vi "PingTestBoard(LC).vi"(0 "COMPORT":refnum<visa-resource-name>, 2 "GuiDir":path, 3 "GlobPaths(t)":bool=TRUE, 5 "error in (no error)":errorcluster, 7 "Mode Select":i32(ring) items=["CW", "DYNAMIC"], 9 "Close Serial(T)":bool, 11 "ExeCommands(T)":bool, 13 "RevC(t)":bool) -> (8 "standard error":string, 10 "standard output":string="Server Status Ok. Received 2048 samples\r\n", 12 "OK?(t)":bool=TRUE, 14 "Run_DMI(t)":bool, 15 "Run_AMInit(t)":bool, 17 "Run -dyn(t)":bool, 19 "error out":errorcluster)   [LabVIEW 2018]
uses:
  Initialize References/Sequence Globals.vi
panel:
  out "ping":string
  out "py_com_port":string
  out "Numeric":i32
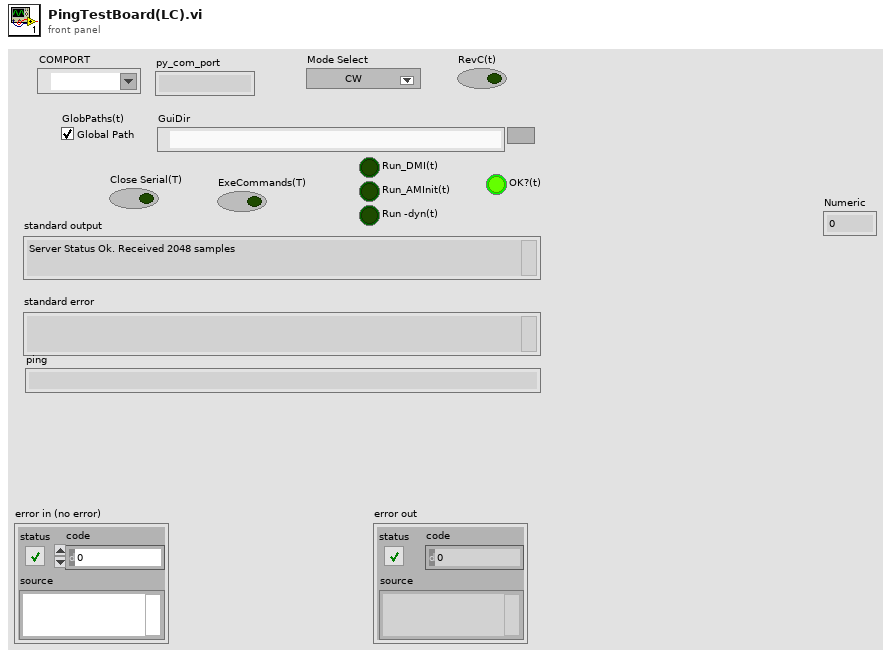
[diagram p1: front panel]
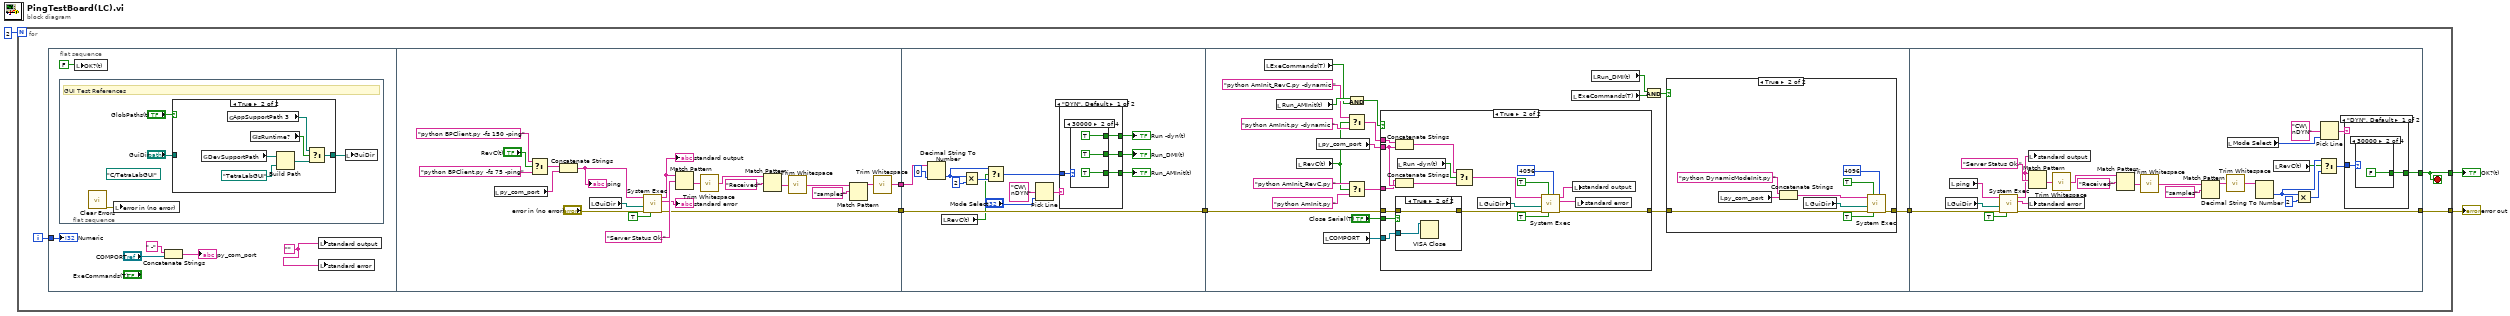
[diagram p0: block diagram]
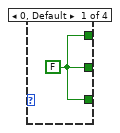
[diagram p3: hidden frame]
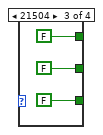
[diagram p4: hidden frame]
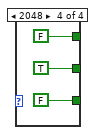
[diagram p5: hidden frame]
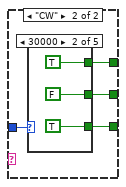
[diagram p6: hidden frame]
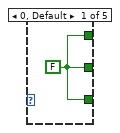
[diagram p7: hidden frame]
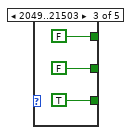
[diagram p8: hidden frame]
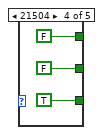
[diagram p9: hidden frame]
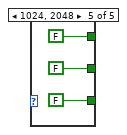
[diagram p10: hidden frame]
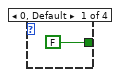
[diagram p14: hidden frame]
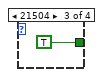
[diagram p15: hidden frame]
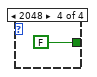
[diagram p16: hidden frame]
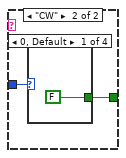
[diagram p17: hidden frame]
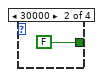
[diagram p18: hidden frame]
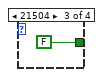
[diagram p19: hidden frame]
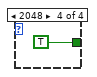
[diagram p20: hidden frame]
diagram:
  n1 = for {
    N: 2 -> [_]
    tunnel: [w6] -> w3
    tunnel: [w5] -> w2
    i -> [w4]
    stop <- w5 stop-if-true
    n2 = flat-sequence {
      tunnel: w4 -> [w12]
      tunnel: [w39] -> w10
      tunnel: [w38] -> w9
      tunnel: w10 -> [w55]
      tunnel: [w58] -> w8
      tunnel: w9 -> [w58]
      tunnel: w8 -> [w112]
      tunnel: [w110] -> w7
      tunnel: [w156] -> w6
      tunnel: w7 -> [w157]
      tunnel: [w153] -> w5
      frame #0 {
        w11 = ""
        n3 = flat-sequence {
          frame #0 {
            (unwired) path "C:/TetraLabGUI" ("PyScript(path)")
            # "GUI Test References"
            n4 = call <vilib>:"Clear Errors.vi"() -> ("error out"=w19:errorcluster)  [unwired: 6 in, 1 out]
            n5 = local write "error in (no error)"(w19) -> ()
            n6 = case shown="True" "GlobPaths(t)" {
              tunnel: [w21 w25] -> w20
              tunnel: "GuiDir" -> [w21 _]
              frame False {
              }
              frame True {
                n7 = global read "Sequence Globals.vi" "DevSupportPath"() -> (w24:path)
                n8 = global read "Sequence Globals.vi" "AppSupportPath 3"() -> (w26:path)
                n9 = global read "Sequence Globals.vi" "IsRuntime?"() -> (w27:bool)
                n10 = Build Path(base path=w24, name or relative path=path "TetraLabGUI" ("PyScript(path)")) -> (appended path=w22:path)
                n11 = Select(t=w26, s=w27, f=w22) -> (s? t:f=w25:path)
              }
            }
            n12 = local write "GuiDir"(w20) -> ()
          }
        }
        n13 = local write "OK?(t)"(FALSE ("OK?(t)")) -> ()
        n14 = Concatenate Strings(" -" ("string"), "COMPORT") -> (→"py_com_port":string)
        n15 = local write "standard output"(w11) -> ()
        n16 = local write "standard error"(w11) -> ()
        "Numeric" <- w12
      }
      frame #1 {
        n17 = local read "py_com_port"() -> (w32:string)
        n18 = Select(t="python BPClient.py -fs 150 -ping" ("command line"), s="RevC(t)", f="python BPClient.py -fs 75 -ping" ("command line")) -> (s? t:f=w31:string)
        n19 = Concatenate Strings(w31, w32) -> (w33:string)
        "ping" <- w33
        n20 = local read "GuiDir"() -> (w34:path)
        n21 = call <vilib>:"System Exec.vi"("run minimized? (F)"=TRUE, "error in (no error)"="error in (no error)", "working directory"=w34, "command line"=w33) -> ("error out"=w38:errorcluster, "standard error"=→"standard error":string, "standard output"=w48:string)  [unwired: 4 in, 1 out]
        "standard output" <- w48
        n22 = Match Pattern(string=w48, regular expression="Server Status Ok.") -> (after substring=w43:string)  [unwired: 1 in, 3 out]
        n23 = call <vilib>:"Trim Whitespace.vi"("string"=w43) -> ("trimmed string"=w44:string)  [unwired: 1 in]
        n24 = Match Pattern(string=w44, regular expression="Received") -> (after substring=w45:string)  [unwired: 1 in, 3 out]
        n25 = call <vilib>:"Trim Whitespace.vi"("string"=w45) -> ("trimmed string"=w47:string)  [unwired: 1 in]
        n26 = Match Pattern(string=w47, regular expression="samples") -> (before substring=w46:string)  [unwired: 1 in, 3 out]
        n27 = call <vilib>:"Trim Whitespace.vi"("string"=w46) -> ("trimmed string"=w39:string)  [unwired: 1 in]
      }
      frame #2 {
        n28 = Decimal String To Number(string=w55, default (0L)=i16 0 ("default (0 I32)")) -> (number=w52:i16)  [unwired: 1 in, 1 out]
        n29 = local read "RevC(t)"() -> (w49:bool)
        n30 = Multiply(x=w52, y=i16 2) -> (x*y=w53:i16)
        n31 = Select(t=w52, s=w49, f=w53) -> (s? t:f=w50:i16)
        n32 = Pick Line(multi-line string="CW\nDYN", line index="Mode Select") -> (output string=w61:string)  [unwired: 1 in]
        n33 = case shown="\"DYN\", Default" w61 {
          tunnel: w50 -> [w66 w80]
          tunnel: [w65 w79] -> w56
          tunnel: [w64 w78] -> w59
          tunnel: [w63 w77] -> w57
          frame "DYN", Default {
            n34 = case shown="30000" w66 {
              tunnel: [w67 TRUE FALSE TRUE] -> w65
              tunnel: [w67 TRUE FALSE FALSE] -> w64
              tunnel: [w67 TRUE FALSE FALSE] -> w63
              frame 0, Default {
                w67 = FALSE
              }
              frame 30000 {
              }
              frame 21504 {
              }
              frame 2048 {
              }
            }
          }
          frame "CW" {
            n35 = case shown="30000" w80 {
              tunnel: [w81 FALSE FALSE FALSE FALSE] -> w79
              tunnel: [w81 TRUE TRUE TRUE FALSE] -> w78
              tunnel: [w81 TRUE FALSE FALSE FALSE] -> w77
              frame 0, Default {
                w81 = FALSE
              }
              frame 30000 {
              }
              frame 2049..21503 {
              }
              frame 21504 {
              }
              frame 1024, 2048 {
              }
            }
          }
        }
        "Run_DMI(t)" <- w56
        "Run_AMInit(t)" <- w59
        "Run -dyn(t)" <- w57
      }
      frame #3 {
        n36 = local read "ExeCommands(T)"() -> (w104:bool)
        n37 = local read "Run_AMInit(t)"() -> (w105:bool)
        n38 = local read "RevC(t)"() -> (w94:bool)
        n39 = local read "py_com_port"() -> (w101:string)
        n40 = local read "COMPORT"() -> (w102:refnum<visa-resource-name>)
        n41 = And(x=w105, y=w104) -> (x .and. y?=w109:bool)
        n42 = Select(t="python AmInit_RevC.py -dynamic " ("command line"), s=w94, f="python AmInit.py -dynamic " ("command line")) -> (s? t:f=w98:string)
        n43 = Select(t="python AmInit_RevC.py " ("command line"), s=w94, f="python AmInit.py " ("command line")) -> (s? t:f=w95:string)
        n44 = case shown="True" w109 {
          tunnel: w112 -> [w123 w136]
          tunnel: [w123 w138] -> w111
          tunnel: w102 -> [_ w134]
          tunnel: "Close Serial(T)" -> [_ w133]
          tunnel: w101 -> [_ w129]
          tunnel: w98 -> [_ w128]
          tunnel: w95 -> [_ w127]
          frame False {
          }
          frame True {
            n45 = Concatenate Strings(w128, w129) -> (w131:string)
            n46 = Concatenate Strings(w127, w129) -> (w130:string)
            n47 = case shown="True" w133 {
              tunnel: w136 -> [w142 w143]
              tunnel: [w142 w143] -> w135
              tunnel: w134 -> [_ w144]
              frame False {
              }
              frame True {
                n48 = VISA Close(VISA resource name=w144) -> ()  [unwired: 1 in, 1 out]
              }
            }
            n49 = local read "Run -dyn(t)"() -> (w137:bool)
            n50 = Select(t=w131, s=w137, f=w130) -> (s? t:f=w126:string)
            n51 = local read "GuiDir"() -> (w132:path)
            n52 = call <vilib>:"System Exec.vi"("expected output size  (4096)"=u32 4096, "run minimized? (F)"=TRUE, "wait until completion? (T)"=TRUE, "error in (no error)"=w135, "working directory"=w132, "command line"=w126) -> ("error out"=w138:errorcluster, "standard error"=w125:string, "standard output"=w124:string)  [unwired: 2 in, 1 out]
            n53 = local write "standard output"(w124) -> ()
            n54 = local write "standard error"(w125) -> ()
          }
        }
        n55 = local read "ExeCommands(T)"() -> (w106:bool)
        n56 = local read "Run_DMI(t)"() -> (w107:bool)
        n57 = And(x=w107, y=w106) -> (x .and. y?=w108:bool)
        n58 = case shown="True" w108 {
          tunnel: [w113 w121] -> w110
          tunnel: w111 -> [w113 w118]
          frame False {
          }
          frame True {
            n59 = local read "py_com_port"() -> (w114:string)
            n60 = Concatenate Strings("python DynamicModeInit.py " ("command line"), w114) -> (w115:string)
            n61 = local read "GuiDir"() -> (w116:path)
            n62 = call <vilib>:"System Exec.vi"("expected output size  (4096)"=u32 4096, "run minimized? (F)"=TRUE, "wait until completion? (T)"=TRUE, "error in (no error)"=w118, "working directory"=w116, "command line"=w115) -> ("error out"=w121:errorcluster)  [unwired: 2 in, 3 out]
          }
        }
      }
      frame #4 {
        n63 = local read "GuiDir"() -> (w152:path)
        n64 = local read "ping"() -> (w145:string)
        n65 = call <vilib>:"System Exec.vi"("run minimized? (F)"=TRUE, "error in (no error)"=w157, "working directory"=w152, "command line"=w145) -> ("error out"=w156:errorcluster, "standard error"=w154:string, "standard output"=w155:string)  [unwired: 4 in, 1 out]
        n66 = local write "standard output"(w155) -> ()
        n67 = Match Pattern(string=w155, regular expression="Server Status Ok.") -> (after substring=w164:string)  [unwired: 1 in, 3 out]
        n68 = local write "standard error"(w154) -> ()
        n69 = call <vilib>:"Trim Whitespace.vi"("string"=w164) -> ("trimmed string"=w165:string)  [unwired: 1 in]
        n70 = Match Pattern(string=w165, regular expression="Received") -> (after substring=w166:string)  [unwired: 1 in, 3 out]
        n71 = call <vilib>:"Trim Whitespace.vi"("string"=w166) -> ("trimmed string"=w168:string)  [unwired: 1 in]
        n72 = Match Pattern(string=w168, regular expression="samples") -> (before substring=w167:string)  [unwired: 1 in, 3 out]
        n73 = call <vilib>:"Trim Whitespace.vi"("string"=w167) -> ("trimmed string"=w151:string)  [unwired: 1 in]
        n74 = local read "Mode Select"() -> (w169:i32)
        n75 = Decimal String To Number(string=w151) -> (number=w148:i32)  [unwired: 2 in, 1 out]
        n76 = local read "RevC(t)"() -> (w146:bool)
        n77 = Multiply(x=w148, y=2) -> (x*y=w149:i32)
        n78 = Select(t=w148, s=w146, f=w149) -> (s? t:f=w150:i32)
        n79 = Pick Line(multi-line string="CW\nDYN", line index=w169) -> (output string=w163:string)  [unwired: 1 in]
        n80 = case shown="\"DYN\", Default" w163 {
          tunnel: w150 -> [w171 w177]
          tunnel: [w170 w176] -> w153
          frame "DYN", Default {
            n81 = case shown="30000" w171 {
              tunnel: [FALSE FALSE TRUE FALSE] -> w170
              frame 0, Default {
              }
              frame 30000 {
              }
              frame 21504 {
              }
              frame 2048 {
              }
            }
          }
          frame "CW" {
            n82 = case shown="0, Default" w177 {
              tunnel: [FALSE FALSE FALSE TRUE] -> w176
              frame 0, Default {
              }
              frame 30000 {
              }
              frame 21504 {
              }
              frame 2048 {
              }
            }
          }
        }
      }
    }
  }
  "error out" <- w3
  "OK?(t)" <- w2
